vi "Build Status.vi"(11 "Git Info":T1) -> (2 "Color":u32(colorbox)=13816530, 3 "Status String":string)   [LabVIEW 2020, in "VolatusGUI.lvlib" / "Git Updater Module.lvclass"]
uses:
  Git Updater Module.lvclass
  Git Info.ctl
  <vilib>/Hampel Software Engineering/Git API/Git API/Controls/GIT-Repository States.ctl
  Git Updater Module.lvclass/Git Updater Module.ctl
  <vilib>/Hampel Software Engineering/Git API/Git API/GIT-api.lvclass
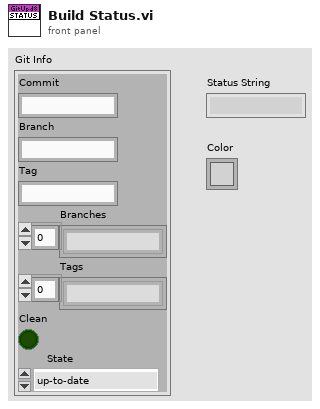
[diagram p1: front panel]
types:
  T1 = typedef "VolatusGUI.lvlib/Git Updater Module.lvclass/Git Info.ctl" = cluster{"Commit":string, "Branch":string, "Tag":string, "Branches":string[], "Tags":string[], "Clean":bool, "State":T2}
  T2 = typedef "GIT-API-for-LabVIEW.lvlib/GIT-api.lvclass/GIT-Repository States.ctl" = enum16{"up-to-date", "behind", "ahead", "diverged", "unpublished", "detached", "unknown"}
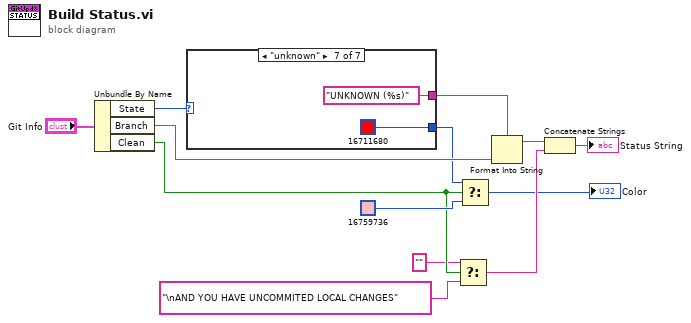
[diagram p0: block diagram]
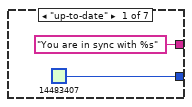
[diagram p2: hidden frame]
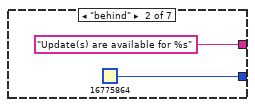
[diagram p3: hidden frame]
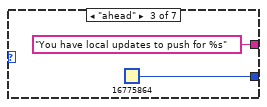
[diagram p4: hidden frame]
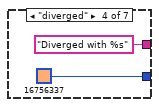
[diagram p5: hidden frame]
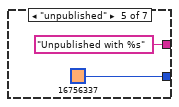
[diagram p6: hidden frame]
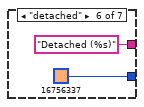
[diagram p7: hidden frame]
diagram:
  n1 = Unbundle By Name("Git Info") -> ("State"=w12:T2, "Branch"=w10:string, "Clean"=w6:bool)
  n2 = case shown="\"unknown\"" w12 {
    tunnel: ["You are in sync with %s" "Update(s) are available for %s" "You have local updates to push for %s" "Diverged with %s" "Unpublished with %s" "Detached (%s)" "UNKNOWN (%s)"] -> w11
    tunnel: [u32 14483407 u32 16775864 u32 16775864 u32 16756337 u32 16756337 u32 16756337 u32 16711680] -> w8
    frame "up-to-date" {
    }
    frame "behind" {
    }
    frame "ahead" {
    }
    frame "diverged" {
    }
    frame "unpublished" {
    }
    frame "detached" {
    }
    frame "unknown" {
    }
  }
  n3 = Select(t="", s=w6, f="\nAND YOU HAVE UNCOMMITED LOCAL CHANGES") -> (s? t:f=w2:string)
  n4 = Select(t=w8, s=w6, f=u32 16759736) -> (s? t:f=→"Color":u32)
  n5 = Format Into String(format string=w11, w10) -> (resulting string=w9:string)  [unwired: 2 in, 1 out]
  n6 = Concatenate Strings(w9, w2) -> (→"Status String":string)
